vi "Find All Tests in Project.vi"(8 "error in (no error)":errorcluster, 10 "Projext Path":path, 11 "LUnit Test Suite In":refnum<class "LUnit Test Suite.lvclass">) -> (0 "error out":errorcluster, 3 "LUnit Test Suite out":refnum<class "LUnit Test Suite.lvclass">)   [LabVIEW 2020, in "Test Finder.lvclass"]
uses:
  Test Finder.lvclass
  LUnit Test Suite.lvclass
  C:/git/astemes-lunit/source/Runnable.lvclass
  Test Finder.lvclass/Test Finder.ctl
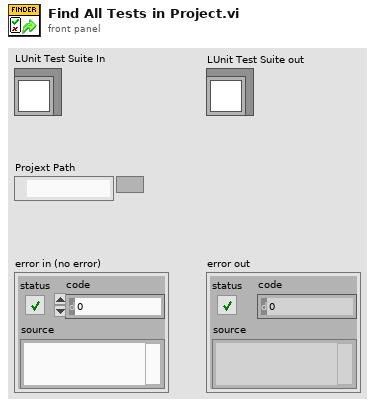
[diagram p1: front panel]
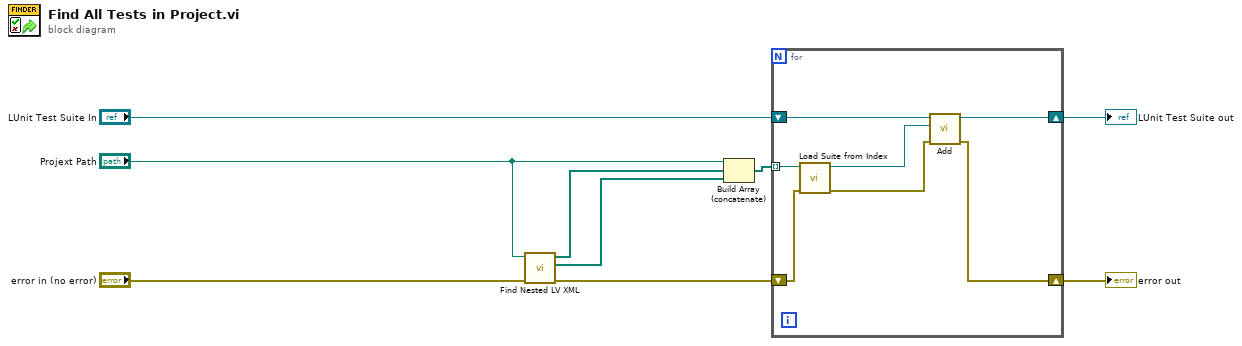
[diagram p0: block diagram]
diagram:
  n1 = call "Find Nested LV XML.vi"("error in (no error)"="error in (no error)", "Projext Path"="Projext Path") -> ("error out"=w4:errorcluster, "lvlibs"=w1:path[], "lvprojs"=w2:path[])  [unwired: 7 in]
  n2 = Build Array (concatenate)("Projext Path", w2, w1) -> (w3:path[])
  n3 = for {
    tunnel: w3 -> [w10] mode=indexing
    shift-right: [w16] -> w9
    shift-left: "LUnit Test Suite In" -> [w14]
    shift-right: [w12] -> w7
    shift-left: w4 -> [w11]
    n4 = call "Load Suite from Index.vi"("error in (no error)"=w11, "Projext Path"=w10) -> ("error out"=w13:errorcluster, "LUnit Test Suite out"=w15:refnum<class "LUnit Test Suite.lvclass">)  [unwired: 8 in]
    n5 = call "Add.vi"("error in (no error)"=w13, "Runnable"=w15, "LUnit Test Suite In"=w14) -> ("error out"=w12:errorcluster, "LUnit Test Suite Out"=w16:refnum<class "LUnit Test Suite.lvclass">)  [unwired: 7 in]
  }
  "LUnit Test Suite out" <- w9
  "error out" <- w7
